vi "TestExec.Script Raw Message to Cluster.vi"(2 "error in":errorcluster, 3 "Message Str":string) -> (0 "error out":errorcluster, 1 "Msg":T1)   [LabVIEW 2017]
uses:
  Controls/TestExec.Script Message.ctl
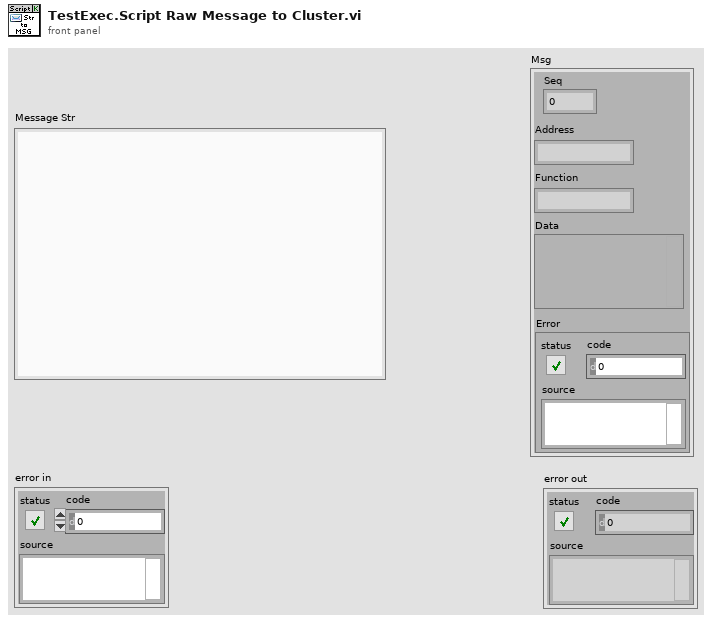
[diagram p1: front panel]
types:
  T1 = typedef "TestExec.Script Message.ctl" = cluster{"Seq":i32, "Address":string, "Function":string, "Data":variant, "Error":errorcluster}
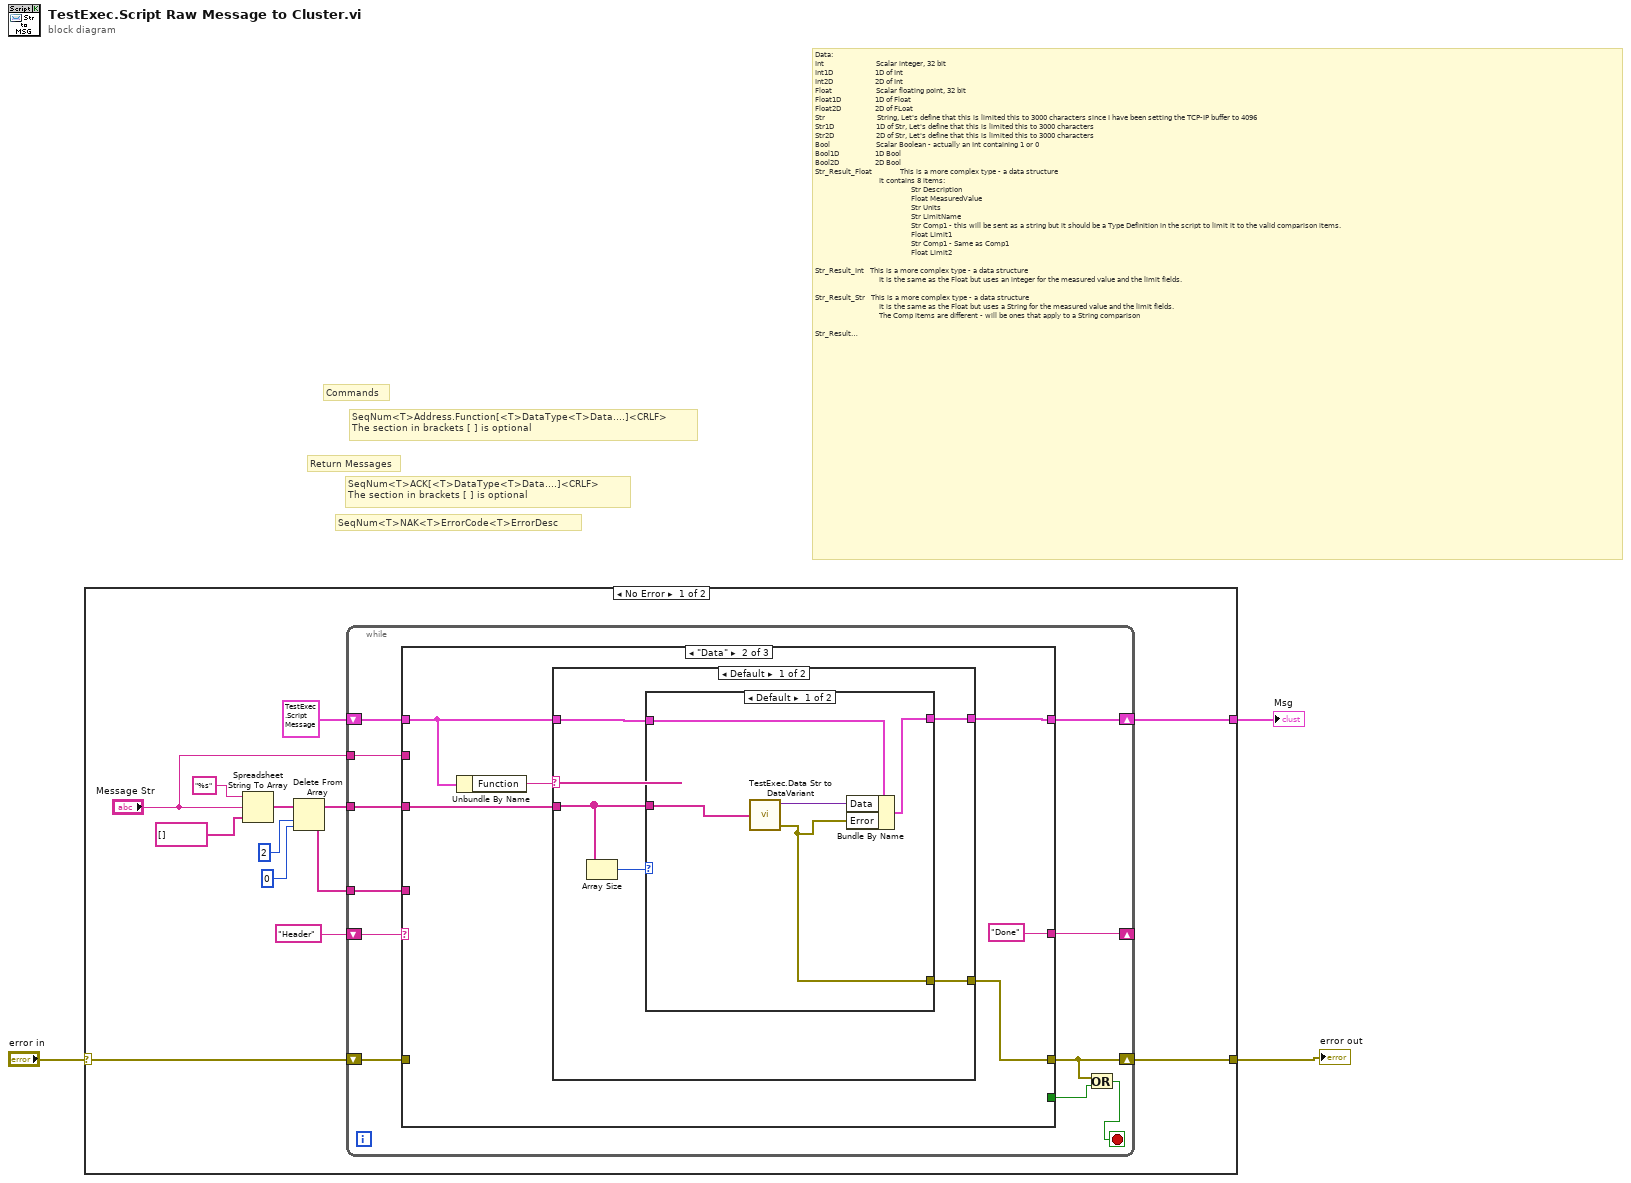
[diagram p0: block diagram]
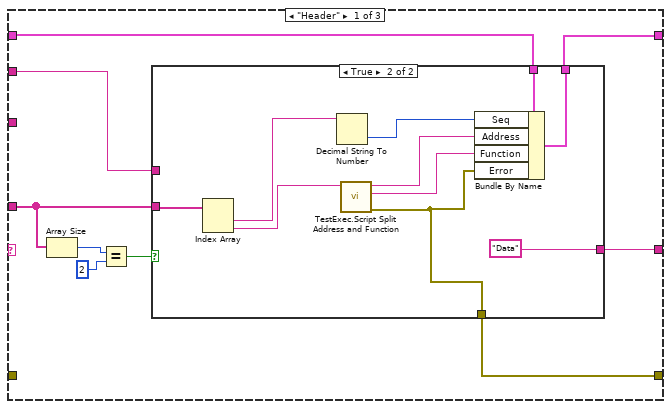
[diagram p2: hidden frame]
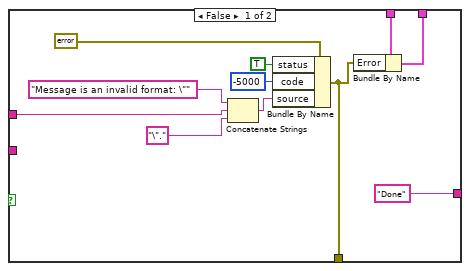
[diagram p3: hidden frame]
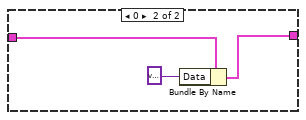
[diagram p4: hidden frame]
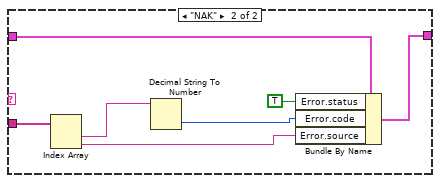
[diagram p5: hidden frame]
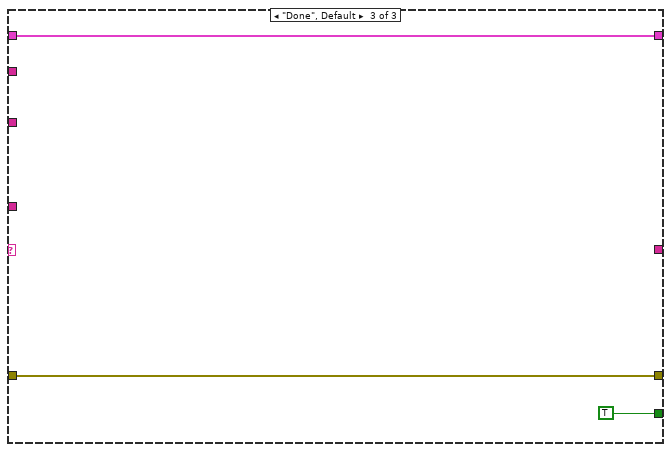
[diagram p6: hidden frame]
diagram:
  # "Data:\nInt                          Scalar integer, 32 bit\nInt1D                     1D of Int\nInt2D                     2D of Int\nFloat                      Scalar floating point, 32 bit\nFloat1D                 1D of Float\nFloat2D                 2D of FLoat\nStr                          String, Let's define that this is limited this to 3000 characters since I have been setting the TCP-IP buffer to 4096\nStr1D                     1D of Str, Let's define that this is limited this to 3000 characters\nStr2D                     2D of Str, Let's define that this is limited this to 3000 characters\nBool                       Scalar Boolean - actually an Int containing 1 or 0\nBool1D                  1D Bool\nBool2D                  2D Bool\nStr_Result_Float              This is a more complex type - a data structure\n                                It contains 8 items:\n                                                Str Description\n                                                Float MeasuredValue\n                                                Str Units\n                                                Str LimitName\n                                                Str Comp1 - this will be sent as a string but it should be a Type Definition in the script to limit it to the valid comparison items.\n                                                Float Limit1\n                                                Str Comp1 - Same as Comp1\n                                                Float Limit2\n \nStr_Result_Int   This is a more complex type - a data structure\n                                It is the same as the Float but uses an integer for the measured value and the limit fields.\n \nStr_Result_Str   This is a more complex type - a data structure\n                                It is the same as the Float but uses a String for the measured value and the limit fields.\n                                The Comp items are different - will be ones that apply to a String comparison\n \nStr_Result_Bool                This is a more complex type - a data structure\n                                It is the same as the Float but uses a Boolean for the measured value and the limit fields.\n                                The Comp items are different - will be ones that apply to a Bool comparison"
  # "Return Messages"
  # "Commands"
  # "SeqNum<T>NAK<T>ErrorCode<T>ErrorDesc"
  # "SeqNum<T>ACK[<T>DataType<T>Data....]<CRLF>  \nThe section in brackets [ ] is optional"
  # "SeqNum<T>Address.Function[<T>DataType<T>Data....]<CRLF>\nThe section in brackets [ ] is optional"
  n1 = case shown="No Error" "error in" {
    selector: "error in" -> [w5 w87]
    tunnel: [w7 _] -> w1
    tunnel: [w6 w87] -> w3
    frame No Error {
      n2 = Spreadsheet String To Array(format string="%s", spreadsheet string="Message Str", array type (2D Dbl)=string[] []) -> (array=w14:string[])  [unwired: 1 in]
      n3 = Delete From Array(array=w14, length=2, index=0) -> (deleted portion=w8:string[], array with subset deleted=w9:string[])
      n4 = while {
        shift-right: [w23] -> w7
        shift-left: T1 {"Seq"=0, "Address"="", "Function"="", "Data"=variant, "Error"={"status"=FALSE, "code"=0, "source"=""}} ("output cluster") -> [w26]
        shift-right: [w20] -> w6
        shift-left: w5 -> [w21]
        tunnel: w9 -> [w25]
        tunnel: w8 -> [w24]
        shift-right: [w22] -> _
        shift-left: "Header" -> [w27]
        tunnel: "Message Str" -> [w17]
        stop <- w18 stop-if-true
        n5 = case shown="\"Data\"" w27 {
          tunnel: w26 -> [w34 w62 w86]
          tunnel: w25 -> [_ w61 _]
          tunnel: w24 -> [w28 _ _]
          tunnel: [w32 w60 w86] -> w23
          tunnel: [w31 "Done" _] -> w22
          tunnel: [w29 w58 w85] -> w20
          tunnel: w21 -> [_ _ w85]
          tunnel: [_ _ TRUE] -> w19
          tunnel: w17 -> [w30 _ _]
          frame "Header" {
            n6 = Array Size(array=w28) -> (size(s)=w35:i32)
            n7 = Equal?(x=w35, y=2) -> (x = y?=w33:bool)
            n8 = case shown="True" w33 {
              tunnel: w34 -> [w47 w56]
              tunnel: [w46 w55] -> w32
              tunnel: ["Done" "Data"] -> w31
              tunnel: w30 -> [w40 _]
              tunnel: [w37 w48] -> w29
              tunnel: w28 -> [_ w54]
              frame False {
                n9 = Concatenate Strings("Message is an invalid format: \"", w40, "\".") -> (w38:string)
                n10 = Bundle By Name(cluster=errorcluster {"status"=FALSE, "code"=0, "source"=""} ("error constant"), "status"=TRUE, "code"=-5000, "source"=w38) -> (w37:errorcluster)
                n11 = Bundle By Name(cluster=w47, "Error"=w37) -> (w46:T1)
              }
              frame True {
                n12 = Index Array(array=w54) -> (element #1=w53:string, element #2=w51:string)  [unwired: 2 in]
                n13 = Decimal String To Number(string=w53) -> (number=w52:i32)  [unwired: 2 in, 1 out]
                n14 = call "TestExec.Script Split Address and Function.vi"("string"=w51) -> ("error out"=w48:errorcluster, "Funct"=w49:string, "Addr"=w50:string)  [unwired: 8 in]
                n15 = Bundle By Name(cluster=w56, "Seq"=w52, "Address"=w50, "Function"=w49, "Error"=w48) -> (w55:T1)
              }
            }
          }
          frame "Data" {
            n16 = Unbundle By Name(w62) -> ("Function"=w63:string)
            n17 = case shown="Default" w63 {
              tunnel: w62 -> [w68 w83]
              tunnel: w61 -> [w65 w82]
              tunnel: [w67 w77] -> w60
              tunnel: [w64 _] -> w58
              frame Default {
                n18 = Array Size(array=w65) -> (size(s)=w66:i32)
                n19 = case shown="Default" w66 {
                  tunnel: w68 -> [w73 w75]
                  tunnel: [w72 w76] -> w67
                  tunnel: w65 -> [w71 _]
                  tunnel: [w69 _] -> w64
                  frame Default {
                    n20 = call "TestExec.Data Str to DataVariant.vi"("DataArray"=w71) -> ("error out"=w69:errorcluster, "Data"=w70:variant)  [unwired: 3 in]
                    n21 = Bundle By Name(cluster=w73, "Data"=w70, "Error"=w69) -> (w72:T1)
                  }
                  frame 0 {
                    n22 = Bundle By Name(cluster=w75, "Data"=variant) -> (w76:T1)
                  }
                }
              }
              frame "NAK" {
                n23 = Index Array(array=w82) -> (element #1=w80:string, element #2=w81:string)  [unwired: 2 in]
                n24 = Decimal String To Number(string=w80) -> (number=w79:i32)  [unwired: 2 in, 1 out]
                n25 = Bundle By Name(cluster=w83, "Error.status"=TRUE, "Error.code"=w79, "Error.source"=w81) -> (w77:T1)
              }
            }
          }
          frame "Done", Default {
          }
        }
        n26 = Or(x=w20, y=w19) -> (x .or. y?=w18:bool)
      }
    }
    frame Error {
    }
  }
  "Msg" <- w1
  "error out" <- w3
